vi "FRCts20_WebMethods_Reports_GET.vi"(11 "httpRequestID":u32) -> ()   [LabVIEW 2014, in "FRCts20_WebMethods.lvlib"]
uses:
  FRCts20_WebMethods.lvlib
  ESP Engine/source/VI Source/FRCts20_EspEngine.lvlib
  Backend/source/VI Source/FRCts20_Backend_API/FRCts20_Backend_API.lvlib
  Backend/source/VI Source/FRCts20_Backend_API/FRCts20_Backend_API_Stats.vi
  ESP Engine/source/VI Source/TypeDefs/FRCts20_EspEngine_RequestPerHour_Line.ctl
  ESP Engine/source/VI Source/TypeDefs/FRCts20_EspEngine_SwUsage_Pie.ctl
  ESP Engine/source/VI Source/TypeDefs/FRCts20_EspEngine_AdvancedComponents_Bar.ctl
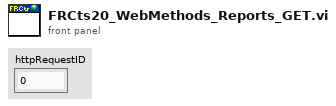
[diagram p1: front panel]
types:
  T1 = typedef "FRCts20_EspEngine.lvlib/FRCts20_EspEngine_SearchBrowser.ctl" = cluster{"Event":cluster{"Event Index":u32, "Event Name":string, "Start Time":timestamp, "End Time":timestamp, "OpenIssues":u8, "IsLive":bool}[], "select-choice-software":string, "select-choice-location":string}
  T2 = cluster{"Event Index":u32, "Event Name":string, "Start Time":timestamp, "End Time":timestamp, "OpenIssues":u8, "IsLive":bool}[]
  T3 = typedef "FRCts20_EspEngine.lvlib/FRCts20_EspEngine_SwUsage_Pie.ctl" = cluster{"Live Event Location":string, "LabVIEW":dbl, "C++":dbl, "Java":dbl, "Other":dbl, "TotalTeams":i32, "TeamsReporting":i32}[]
  T4 = typedef "FRCts20_EspEngine.lvlib/FRCts20_EspEngine_RequestPerHour_Line.ctl" = cluster{"StartDate":cluster{"Year":i32, "Month":i32, "Day":i32}, "Events":cluster{"Location":string, "Requests":i32[]}[]}
  T5 = typedef "FRCts20_EspEngine.lvlib/FRCts20_EspEngine_AdvancedComponents_Bar.ctl" = cluster{"CAN":i32, "Vision":i32, "Kinect":i32}
  T6 = cluster{"SW Usage Pies":T3, "RequestsPerHour":T4, "Advanced Components":T5}
  T7 = typedef "FRCts20_Backend_API.lvlib/FRCts20_Backend_API_Stats.ctl" = cluster{"RequestsPerHour":T4, "SW Usage Pies":T3, "Advanced Components":T5, "APIReturn":string}
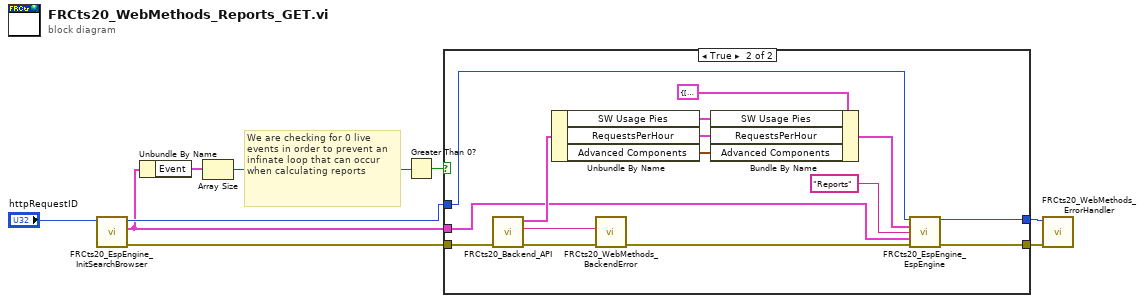
[diagram p0: block diagram]
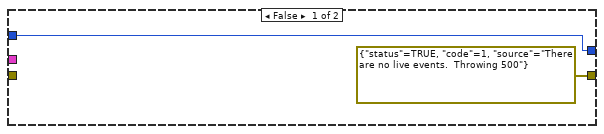
[diagram p2: hidden frame]
diagram:
  # "We are checking for 0 live events in order to prevent an infinate loop that can occur when calculating reports"
  n1 = call "FRCts20_EspEngine_InitSearchBrowser.vi"("httpRequestID"="httpRequestID") -> ("error out"=w7:errorcluster, "SearchBrowser"=w4:T1, "httpRequestID out"=w5:u32)  [unwired: 8 in]
  n2 = Unbundle By Name(w4) -> ("Event"=w3:T2)
  n3 = Array Size(array=w3) -> (size(s)=w2:i32)
  n4 = Greater Than 0?(x=w2) -> (x > 0?=w1:bool)
  n5 = case shown="True" w1 {
    tunnel: [errorcluster {"status"=TRUE, "code"=1, "source"="There are no live events.  Throwing 500"} ("error out") w26] -> w9
    tunnel: [w10 w25] -> w8
    tunnel: w7 -> [_ w14]
    tunnel: w5 -> [w10 w13]
    tunnel: w4 -> [_ w12]
    frame False {
    }
    frame True {
      n6 = call-poly "FRCts20_Backend_API.vi"("error in (no error)"=w14) -> ("error out"=w24:errorcluster, "Status"=w23:string, "Statistics Out"=w21:T7)  [unwired: 8 in]
      n7 = Unbundle By Name(w21) -> ("SW Usage Pies"=w19:T3, "RequestsPerHour"=w18:T4, "Advanced Components"=w15:T5)
      n8 = call "FRCts20_WebMethods_BackendError.vi"("error in (no error)"=w24, "Status"=w23) -> ("error out"=w20:errorcluster)  [unwired: 8 in, 1 out]
      n9 = Bundle By Name(cluster=T6 {"SW Usage Pies"=[], "RequestsPerHour"={"StartDate"={"Year"=0, "Month"=0, "Day"=0}, "Events"=[]}, "Advanced Components"={"CAN"=0, "Vision"=0, "Kinect"=0}} ("output cluster"), "SW Usage Pies"=w19, "RequestsPerHour"=w18, "Advanced Components"=w15) -> (w17:T6)
      n10 = call "FRCts20_EspEngine_EspEngine.vi"("httpRequestID"=w13, "Cluster"=w17, "Page"="Reports", "SearchBrowser"=w12, "error in (no error)"=w20) -> ("httpRequestID out"=w25:u32, "error out"=w26:errorcluster)  [unwired: 9 in]
    }
  }
  n11 = call "FRCts20_WebMethods_ErrorHandler.vi"("error in"=w9, "httpRequestID"=w8) -> ()  [unwired: 9 in, 1 out]
